vi "Detect.vi"(8 "error in (no error)":errorcluster, 11 "Software Lock-in in":refnum<class "Software Lock-in.lvclass">) -> (0 "error out":errorcluster, 2 "Finished":bool, 3 "Software Lock-in out":refnum<class "Software Lock-in.lvclass">)   [LabVIEW 2015, in "Software Lock-in.lvclass"]
uses:
  Software Lock-in.lvclass
  Software Lock-in.lvclass/Software Lock-in.ctl
  <vilib>/Analysis/2dsp.llb/Decimate (continuous, CDB).vi
  <vilib>/Analysis/NI_AALPro.lvlib
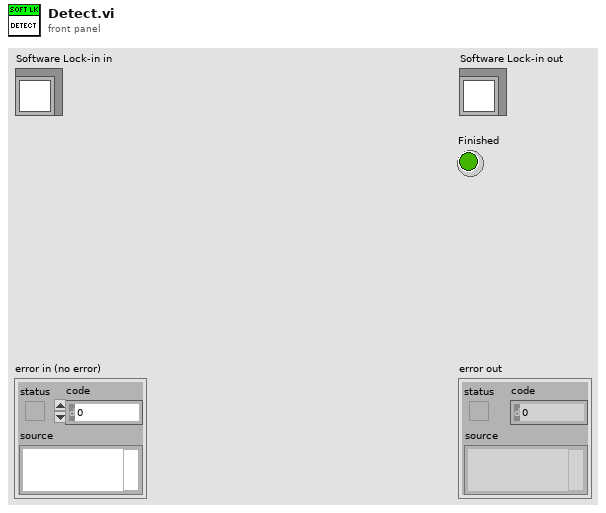
[diagram p1: front panel]
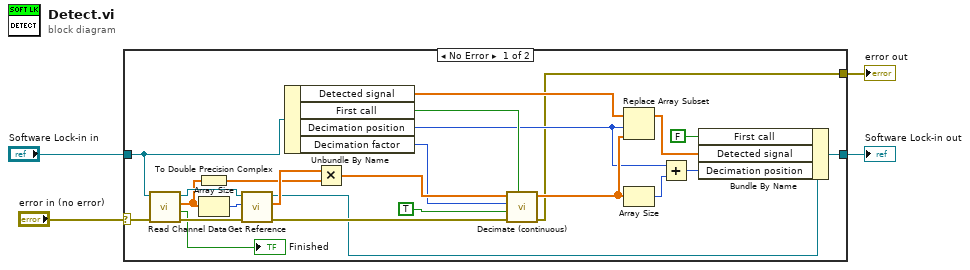
[diagram p0: block diagram]
diagram:
  n1 = case shown="No Error" "error in (no error)" {
    selector: "error in (no error)" -> [w7 w30]
    tunnel: [w6 w30] -> w3
    tunnel: [w19 w29] -> w1
    tunnel: "Software Lock-in in" -> [w21 w29]
    frame No Error {
      n2 = call-dynamic "Read Channel Data.vi"("error in (no error)"=w7, "Software Lock-in in"=w21) -> ("error out"=w26:errorcluster, "Finished"=→"Finished":bool, "Data"=w24:dbl[], "Software Lock-in out"=w28:refnum<class "Software Lock-in.lvclass">)  [unwired: 6 in]
      n3 = To Double Precision Complex(1:w24) -> (0:w23:cdb[])
      n4 = Array Size(array=w24) -> (size(s)=w27:i32)
      n5 = call-dynamic "Get Reference.vi"("error in (no error)"=w26, "Samples"=w27, "Software Lock-in in"=w28) -> ("error out"=w17:errorcluster, "Reference"=w25:cdb[], "Software Lock-in out"=w8:refnum<class "Software Lock-in.lvclass">)  [unwired: 6 in]
      n6 = Unbundle By Name(w21) -> ("Detected signal"=w14:cdb[], "First call"=w20:bool, "Decimation position"=w11:i32, "Decimation factor"=w16:i32)
      n7 = Multiply(x=w25, y=w23) -> (x*y=w22:cdb[])
      n8 = call-poly <vilib>:"Decimate (continuous).vi"("reset"=w20, "error in (no error)"=w17, "averaging"=TRUE, "decimating factor"=w16, "X"=w22) -> ("error out"=w6:errorcluster, "Decimated Array"=w12:cdb[])  [unwired: 5 in]
      n9 = Replace Array Subset(array=w14, new element=w12, index=w11) -> (w13:cdb[])
      n10 = Array Size(array=w12) -> (size(s)=w10:i32)
      n11 = Add(x=w11, y=w10) -> (x+y=w9:i32)
      n12 = Bundle By Name(cluster=w8, "First call"=FALSE, "Detected signal"=w13, "Decimation position"=w9) -> (w19:refnum<class "Software Lock-in.lvclass">)
    }
    frame Error {
    }
  }
  "error out" <- w3
  "Software Lock-in out" <- w1
